vi "LCD Servo Home Call.vi"(8 "error in":errorcluster, 10 "Enable(T)/Dissable":bool) -> (0 "error out":errorcluster)   [LabVIEW 2015]
uses:
  Galobal variable_TI.vi
  Project Setup/Globle Variable/GR_Servo.vi
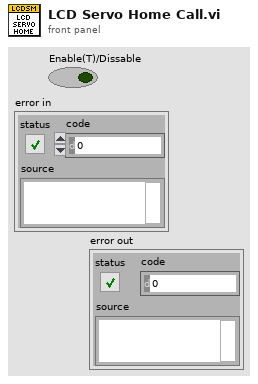
[diagram p1: front panel]
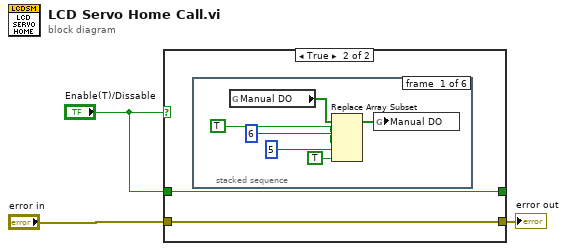
[diagram p0: block diagram]
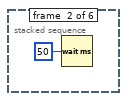
[diagram p3: hidden frame]
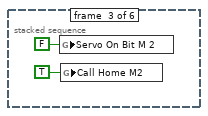
[diagram p4: hidden frame]
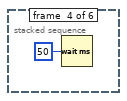
[diagram p5: hidden frame]
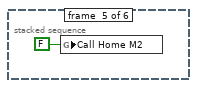
[diagram p6: hidden frame]
diagram:
  n1 = case shown="True" "Enable(T)/Dissable" {
    tunnel: [_ w6] -> _
    tunnel: "Enable(T)/Dissable" -> [_ w6]
    tunnel: [w4 w5] -> w1
    tunnel: "error in" -> [w4 w5]
    frame False {
    }
    frame True {
      n2 = stacked-sequence {
        frame #0 {
          n3 = global read "Galobal variable_TI.vi" "Manual DO"() -> (w12:bool[])
          n4 = Replace Array Subset(array=w12, new element #1=TRUE, index #1=6 ("index"), new element #2=TRUE ("new element/subarray"), index #2=5 ("index")) -> (w9:bool[])
          n5 = global write "Galobal variable_TI.vi" "Manual DO"(w9) -> ()
        }
        frame #1 {
          n6 = Wait (ms)(milliseconds to wait=u32 50) -> ()  [unwired: 1 out]
        }
        frame #2 {
          n7 = global write "GR_Servo.vi" "Servo On Bit M 2"(FALSE ("Servo On Bit")) -> ()
          n8 = global write "Galobal variable_TI.vi" "Call Home M2"(TRUE ("Call Home M1")) -> ()
        }
        frame #3 {
          n9 = Wait (ms)(milliseconds to wait=u32 50) -> ()  [unwired: 1 out]
        }
        frame #4 {
          n10 = global write "Galobal variable_TI.vi" "Call Home M2"(FALSE ("Call Home M1")) -> ()
        }
        frame #5 {
        }
      }
    }
  }
  "error out" <- w1
